vi "MultiChannnel_With_Origin_init.vi"() -> ()   [LabVIEW 2024]
uses:
  <vilib>/DAQmx/read.llb/DAQmx Read (Analog 1D Wfm NChan NSamp).vi
  <vilib>/Analysis/baseanly.llb/Mean (DBL).vi
  <vilib>/DAQmx/create/channels.llb/DAQmx Create Channel (AI-Voltage-Basic).vi
  <vilib>/DAQmx/configure/timing.llb/DAQmx Timing (Sample Clock).vi
  <vilib>/DAQmx/miscellaneous.llb/DAQmx Fill In Error Info.vi
  <vilib>/Waveform/WDTOps.llb/WDT Index Channel DBL.vi
  <vilib>/Analysis/NI_AALBase.lvlib
panel:
  in  "StopAll":bool
  out "Numeric":i32
  out "Ch3 Origin":dbl
  out "Ch2 Origin":dbl
  out "Ch1 Origin":dbl
  out "appended array":dbl[][](array[numeric])
  out "Y 3":dbl[](array[numeric])
  out "Y 2":dbl[](array[numeric])
  out "Y":dbl[](array[numeric])
  in  "Get Orogin":bool
  out "Waveform Graph":waveform(dbl)[](graph)
  in  "samples per channel":i32=500
  in  "sample mode":i32(ring)=10123 items=["Continuous Samples"=10123, "Finite Samples"=10178, "Hardware Timed Single Point"=12522]
  in  "rate":dbl=1000.0 format="%0.2f"
  in  "physical channels":tag="Dev2/ai0:2"
  # "Phy Channel -> Set to 0-2\nRate 1000Hz\nSampleMode  -> Contenious Sampling\nSample per Channel -> 100"
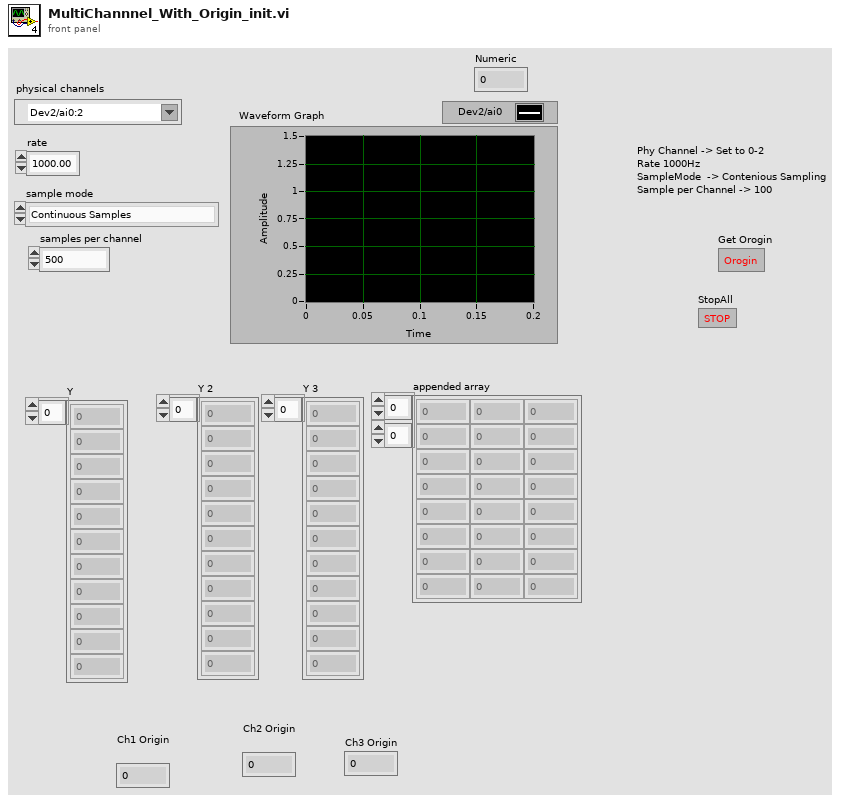
[diagram p1: front panel]
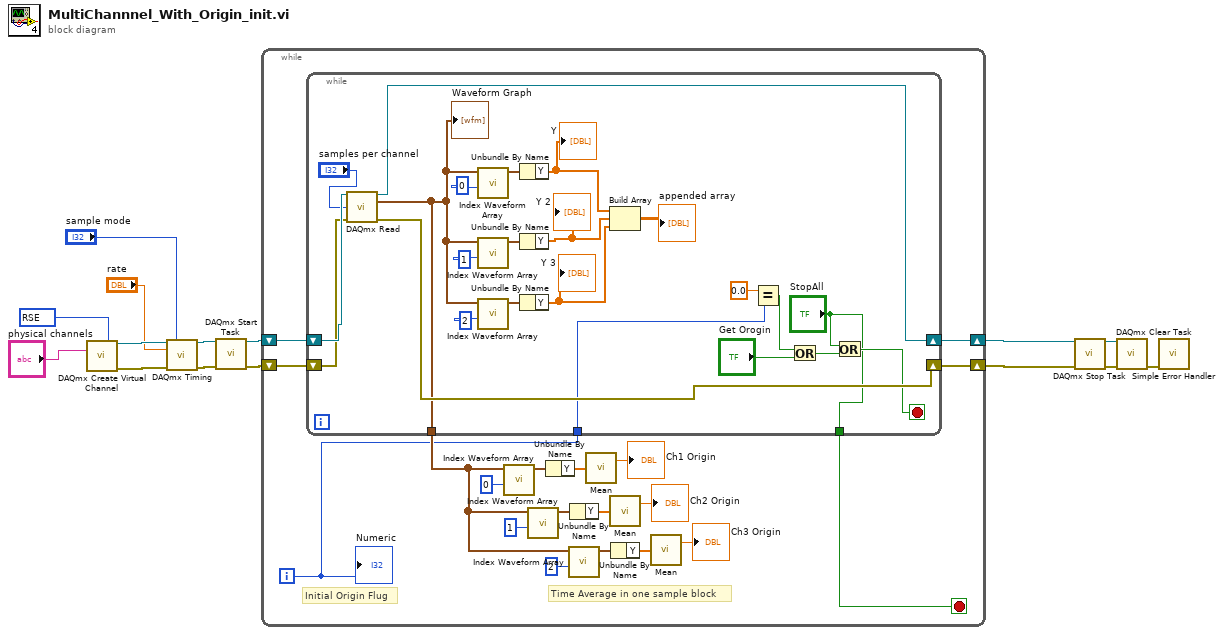
[diagram p0: block diagram]
diagram:
  w1 = 10083 items=["Default"=-1, "RSE"=10083, "NRSE"=10078, "Differential"=10106, "Pseudodifferential"=12529] ("input terminal configuration")
  n1 = call-poly <vilib>:"DAQmx Create Virtual Channel.vi"("input terminal configuration"=w1, "physical channels"="physical channels") -> ("task out"=w7:refnum<k21>, "error out"=w6:errorcluster)  [unwired: 12 in]
  n2 = call-poly <vilib>:"DAQmx Timing.vi"("task/channels in"=w7, "sample mode"="sample mode", "rate"="rate", "error in"=w6) -> ("task out"=w5:refnum<k21>, "error out"=w4:errorcluster)  [unwired: 10 in]
  n3 = call <vilib>:"DAQmx Start Task.vi"("task/channels in"=w5, "error in"=w4) -> ("task out"=w14:refnum<k21>, "error out"=w13:errorcluster)  [unwired: 12 in]
  n4 = while {
    shift-right: [w31] -> w11
    shift-left: w14 -> [w34]
    shift-right: [w32] -> w12
    shift-left: w13 -> [w33]
    i -> [w22]
    stop <- w23 stop-if-true
    # "Time Average in one sample block"
    # "Initial Origin Flug"
    n5 = while {
      shift-right: [w54] -> w31
      shift-left: w34 -> [w57]
      shift-right: [w55] -> w32
      shift-left: w33 -> [w56]
      tunnel: [w42] -> w27
      tunnel: ["StopAll"] -> w23
      tunnel: w22 -> [w38]
      stop <- w41 stop-if-true
      n6 = call-poly <vilib>:"DAQmx Read.vi"("task/channels in"=w57, "number of samples per channel"="samples per channel", "error in"=w56) -> ("task out"=w54:refnum<k21>, "data"=w42:waveform(dbl)[], "error out"=w55:errorcluster)  [unwired: 10 in]
      "Waveform Graph" <- w42
      n7 = call-poly <vilib>:"Index Waveform Array.vi"("index"=0, "waveform array"=w42) -> ("waveform"=w51:waveform(dbl))  [unwired: 8 in, 1 out]
      n8 = call-poly <vilib>:"Index Waveform Array.vi"("index"=1, "waveform array"=w42) -> ("waveform"=w49:waveform(dbl))  [unwired: 8 in, 1 out]
      n9 = call-poly <vilib>:"Index Waveform Array.vi"("index"=2, "waveform array"=w42) -> ("waveform"=w47:waveform(dbl))  [unwired: 8 in, 1 out]
      n10 = Unbundle By Name(w51) -> ("Y"=w46:dbl[])
      "Y" <- w46
      n11 = Unbundle By Name(w49) -> ("Y"=w45:dbl[])
      "Y 2" <- w45
      n12 = Unbundle By Name(w47) -> ("Y"=w44:dbl[])
      "Y 3" <- w44
      n13 = Build Array(w46, w45, w44) -> (→"appended array":dbl[][])
      n14 = Equal?(x=0.0, y=w38) -> (x = y?=w37:bool)
      n15 = Or(x=w37, y="Get Orogin") -> (x .or. y?=w35:bool)
      n16 = Or(x="StopAll", y=w35) -> (x .or. y?=w41:bool)
    }
    n17 = call-poly <vilib>:"Index Waveform Array.vi"("index"=0, "waveform array"=w27) -> ("waveform"=w30:waveform(dbl))  [unwired: 8 in, 1 out]
    n18 = call-poly <vilib>:"Index Waveform Array.vi"("index"=1, "waveform array"=w27) -> ("waveform"=w29:waveform(dbl))  [unwired: 8 in, 1 out]
    n19 = Unbundle By Name(w30) -> ("Y"=w20:dbl[])
    n20 = call-poly <vilib>:"Index Waveform Array.vi"("index"=2, "waveform array"=w27) -> ("waveform"=w28:waveform(dbl))  [unwired: 8 in, 1 out]
    n21 = Unbundle By Name(w29) -> ("Y"=w19:dbl[])
    n22 = call-poly <vilib>:"Mean.vi"("X"=w20) -> ("mean"=→"Ch1 Origin":dbl)  [unwired: 1 out]
    n23 = call-poly <vilib>:"Mean.vi"("X"=w19) -> ("mean"=→"Ch2 Origin":dbl)  [unwired: 1 out]
    n24 = Unbundle By Name(w28) -> ("Y"=w18:dbl[])
    n25 = call-poly <vilib>:"Mean.vi"("X"=w18) -> ("mean"=→"Ch3 Origin":dbl)  [unwired: 1 out]
    "Numeric" <- w22
  }
  n26 = call <vilib>:"DAQmx Stop Task.vi"("task/channels in"=w11, "error in"=w12) -> ("task out"=w9:refnum<k21>, "error out"=w10:errorcluster)  [unwired: 12 in]
  n27 = call <vilib>:"DAQmx Clear Task.vi"("task in"=w9, "error in"=w10) -> ("error out"=w8:errorcluster)  [unwired: 13 in]
  n28 = call <vilib>:"Simple Error Handler.vi"("error in (no error)"=w8) -> ()  [unwired: 4 in, 5 out]
